vi "Launch Test Instr.vi"(0 "Controller in":refnum<class "Controller.lvclass">, 1 "PAS Data":refnum<class "PAS Data.lvclass">=refnum, 5 "error in (no error)":errorcluster) -> (14 "Controller out":refnum<class "Controller.lvclass">, 15 "Boolean":bool, 19 "error out":errorcluster)   [LabVIEW 2014, in "Controller.lvlib" / "Controller.lvclass"]
uses:
  Controller.lvclass
  PAS/Instrument/ePAS.lvclass
  CRDS/Main/eCRDS.lvclass
  <userlib>/_Session Fwk/Session - Root.lvclass
  FPGA/Session/Exscalabar FPGA.lvclass
  Instr Actor/Messages/Send PAS Data MSG/Send PAS Data MSG.lvclass
  Instr Actor/Messages/Send CRD Data MSG/Send CRD Data.lvclass
  Instr Actor/Instr Actor.lvclass
  <vilib>/ActorFramework/Actor/Actor.lvclass
  reusable/PAS/Data/Main/PAS Data.lvclass
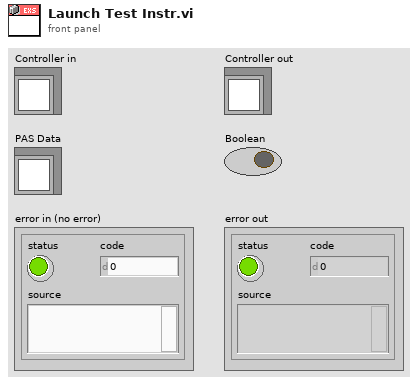
[diagram p1: front panel]
types:
  T1 = typedef "Session - Root.lvclass/Session Handle.ctl" = refnum<data-value>
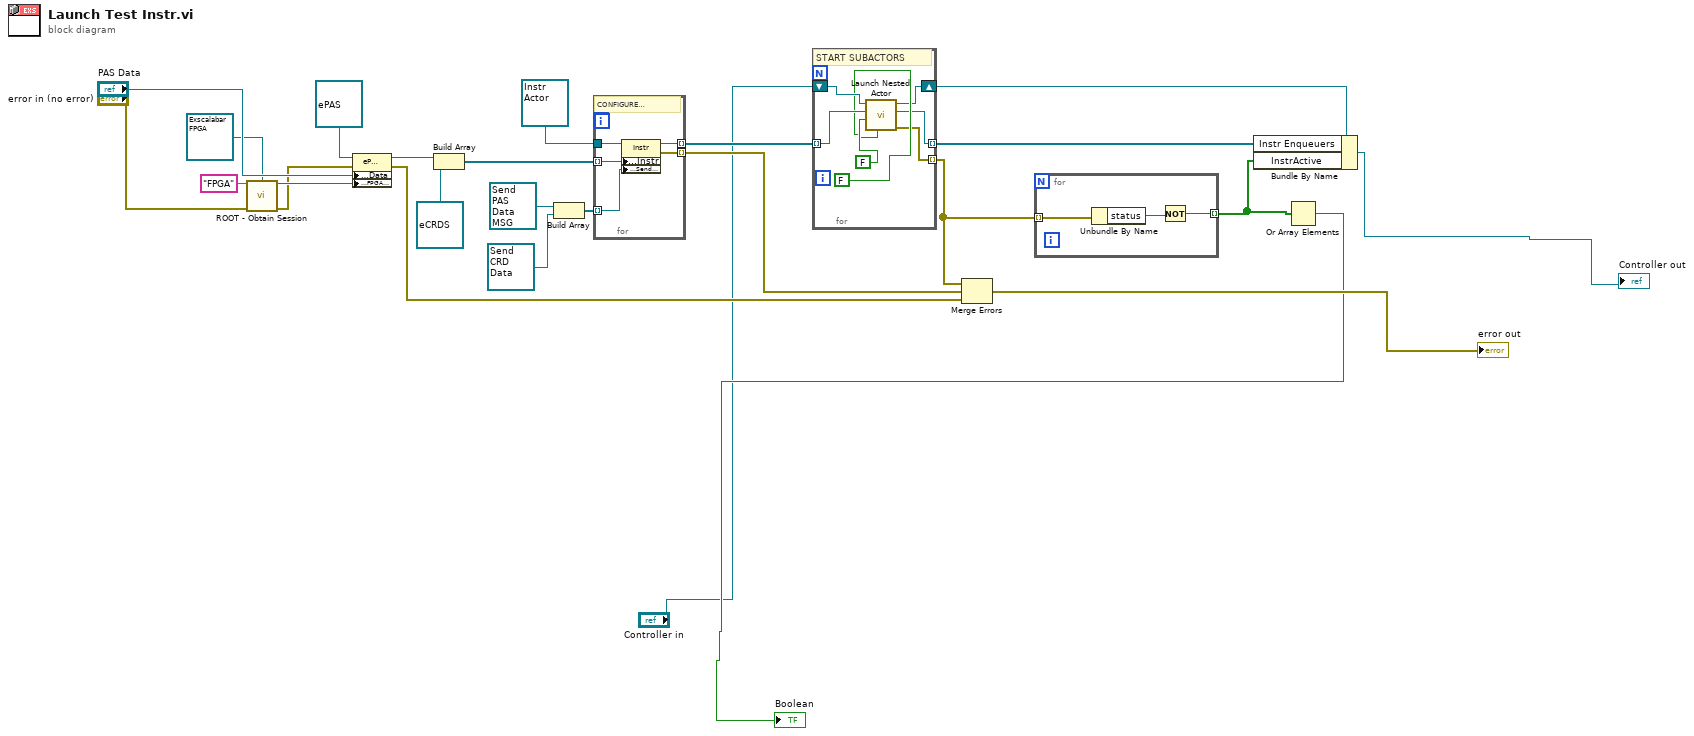
[diagram p0: block diagram]
diagram:
  n1 = call <userlib>:"ROOT - Obtain Session.vi"("Session Name ()"="FPGA", "OBJ - Session"=refnum<class "Exscalabar FPGA.lvclass"> refnum ("Ex FPGA"), "error in (no error)"="error in (no error)") -> ("Session Handle"=w21:T1, "error out"=w10:errorcluster)  [unwired: 10 in, 1 out]
  n2 = property class="ePAS.lvclass"(reference=refnum<class "ePAS.lvclass"> refnum ("ePAS.lvclass"), error in=w10, "Accessors:Data"="PAS Data", "Accessors:FPGA Session"=w21) -> (reference out=w11:refnum<class "ePAS.lvclass">, error out=w18:errorcluster)
  n3 = Build Array(w11, refnum<class "eCRDS.lvclass"> refnum ("eCRDS")) -> (w17:refnum<class>[])
  n4 = Build Array(refnum<class "Send PAS Data MSG.lvclass"> refnum ("Instrument Lib:Send PAS Data"), refnum<class "Send CRD Data.lvclass"> refnum ("Instrument Lib:Send CRD Data")) -> (w7:refnum<class>[])
  n5 = for {
    tunnel: w17 -> [w27] mode=indexing
    tunnel: [w29] -> w19 mode=indexing
    tunnel: [w30] -> w16 mode=indexing
    tunnel: w7 -> [w28] mode=indexing
    tunnel: refnum<class "Instr Actor.lvclass"> refnum ("Instrument Lib:Instr") -> [w26]
    # "CONFIGURE INSTRUMENTS FOR OPERATION"
    n6 = property class="Instr"(reference=w26, "Accessors:Instr"=w27, "Accessors:Send Data MSG"=w28) -> (reference out=w30:refnum<class "Instr Actor.lvclass">, error out=w29:errorcluster)  [unwired: 1 in]
  }
  n7 = for {
    tunnel: w16 -> [w36] mode=indexing
    shift-right: [w33] -> w20
    shift-left: "Controller in" -> [w37]
    tunnel: [w31] -> w23 mode=indexing
    tunnel: [w32] -> w24 mode=indexing
    # "START SUBACTORS"
    n8 = call <vilib>:"Launch Nested Actor.vi"("Open Actor Core front panel? (F)"=FALSE, "Auto-stop? (T)"=FALSE, "Nested Actor"=w36, "Caller Actor in"=w37) -> ("error out"=w32:errorcluster, "Nested Actor's Enqueuer"=w31:refnum<class "Message Enqueuer.lvclass">, "Caller Actor out"=w33:refnum<class "Controller.lvclass">)  [unwired: 5 in]
  }
  n9 = Merge Errors(w24, w19, w18) -> (→"error out":errorcluster)
  n10 = for {
    tunnel: w24 -> [w40] mode=indexing
    tunnel: [w38] -> w25 mode=indexing
    n11 = Unbundle By Name(w40) -> ("status"=w39:bool)
    n12 = Not(x=w39) -> (.not. x?=w38:bool)
  }
  n13 = Bundle By Name(cluster=w20, "Instr Enqueuers"=w23, "InstrActive"=w25) -> (→"Controller out":refnum<class "Controller.lvclass">)
  n14 = Or Array Elements(Boolean array=w25) -> (logical OR=→"Boolean":bool)
